vi "HEWH Rate Total End.vi"(0 "Sub Array End Index in":i32, 1 "Rate":dbl[](array[numeric]), 2 "Total":dbl[](array[numeric]), 11 "error in (no error)":errorcluster) -> (4 "Highest Volume Index":i32, 15 "error out":errorcluster)   [LabVIEW 2023]
panel:
  out "element":dbl
  out "Rate Out (Debug)":dbl[](array[numeric])
  out "Total Out (Debug)":dbl[](array[numeric])
  out "Rate Sub Reversed":dbl[](array[numeric])
  out "Total Sub\nReversed":dbl[](array[numeric])
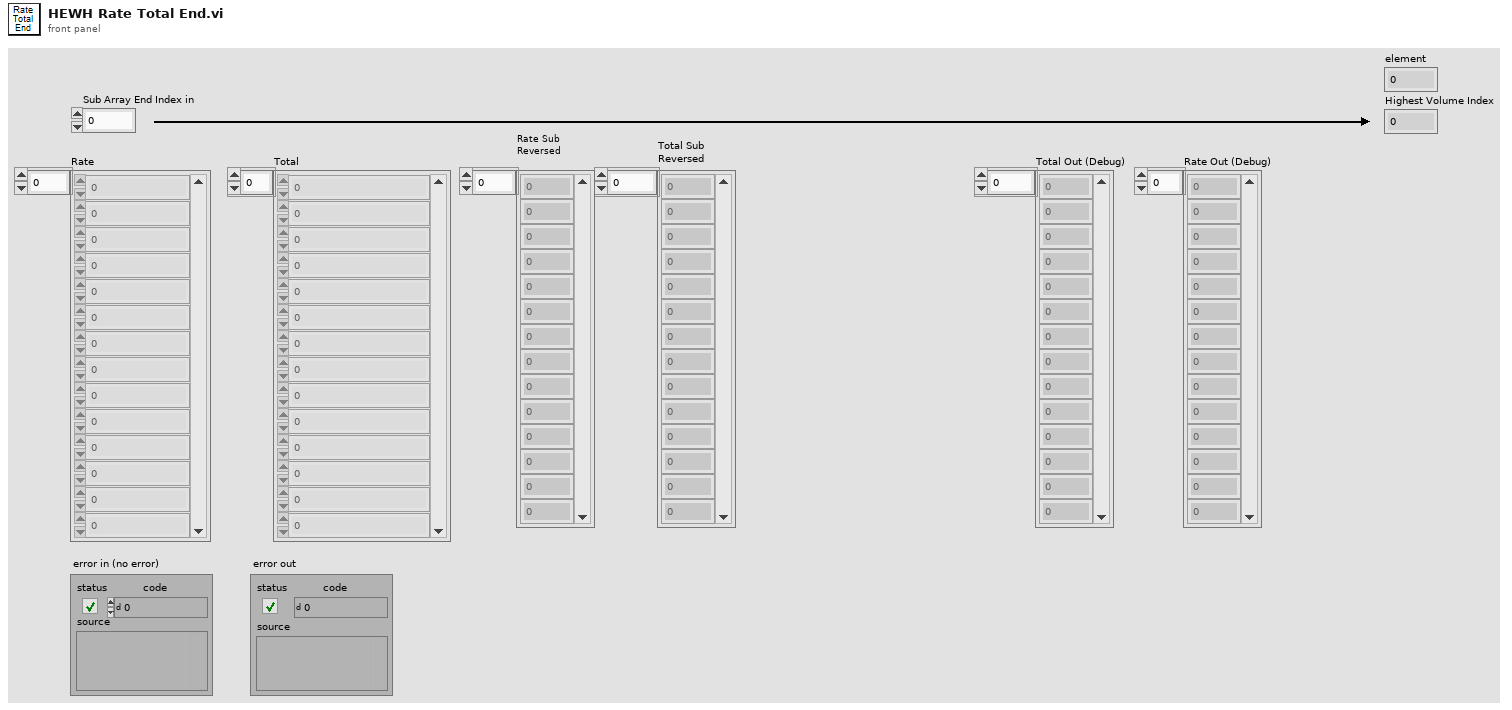
[diagram p1: front panel]
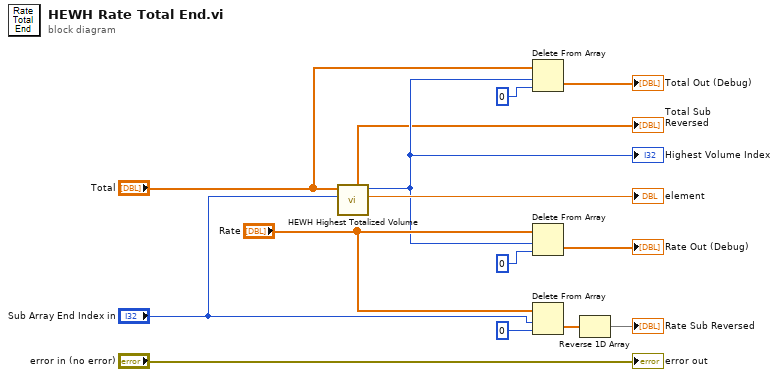
[diagram p0: block diagram]
diagram:
  n1 = call "HEWH Highest Totalized Volume.vi"("Sub Array End Index in"="Sub Array End Index in", "Total in"="Total") -> ("Highest Totalized Volume (gal)"=→"element":dbl, "Sub Array Out"=w3:i32, "Total Sub\nReversed"=→"Total Sub\nReversed":dbl[])  [unwired: 7 in]
  "Highest Volume Index" <- w3
  n2 = Delete From Array(array="Total", length=w3, index=0) -> (deleted portion=→"Total Out (Debug)":dbl[])  [unwired: 1 out]
  n3 = Delete From Array(array="Rate", length=w3, index=0) -> (deleted portion=→"Rate Out (Debug)":dbl[])  [unwired: 1 out]
  n4 = Delete From Array(array="Rate", length="Sub Array End Index in", index=0) -> (deleted portion=w13:dbl[])  [unwired: 1 out]
  n5 = Reverse 1D Array(array=w13) -> (reversed array=→"Rate Sub Reversed":dbl[])
  "error out" <- "error in (no error)"
